vi "POST (File).vi"(6 "timeout":i32=10000, 7 "output file":path, 8 "error in":errorcluster, 9 "file":path, 10 "url":string, 11 "http-method in":refnum<class "REST Client.lvclass">) -> (0 "error out":errorcluster, 2 "response":refnum<class "response.lvclass">, 3 "http-method out":refnum<class "REST Client.lvclass">)   [LabVIEW 2020, in "REST Client.lvlib" / "REST Client.lvclass"]
uses:
  REST Client.lvclass
  response/response.lvclass
  http-client/http-client.lvclass
  REST Client.lvclass/REST Client.ctl
  http.lvlib
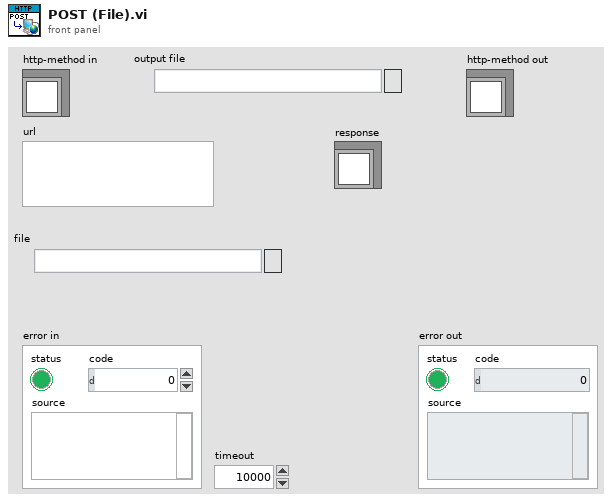
[diagram p1: front panel]
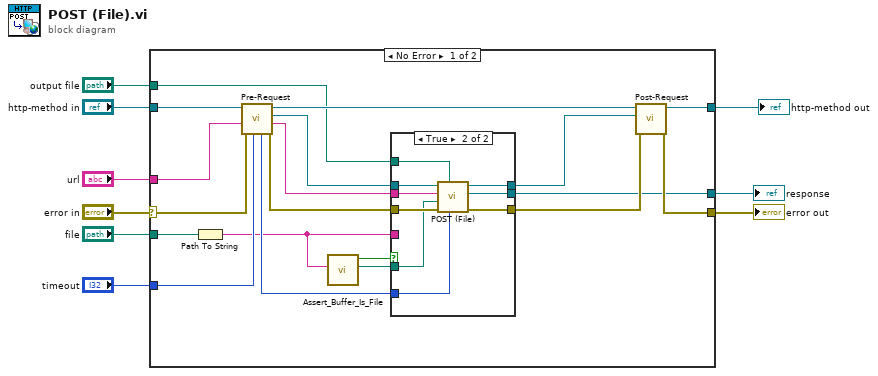
[diagram p0: block diagram]
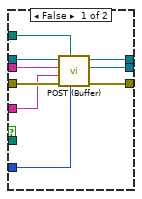
[diagram p2: hidden frame]
diagram:
  n1 = case shown="No Error" "error in" {
    selector: "error in" -> [w27 w48]
    tunnel: [w24 w48] -> w7
    tunnel: [w25 w47] -> w8
    tunnel: "http-method in" -> [w26 w47]
    tunnel: "url" -> [w22 _]
    tunnel: "timeout" -> [w21 _]
    tunnel: "output file" -> [w18 _]
    tunnel: "file" -> [w23 _]
    tunnel: [w10 _] -> w1
    frame No Error {
      n2 = Path To String(path=w23) -> (string=w14:string)
      n3 = call "Pre-Request.vi"("timeout"=w21, "error in (no error)"=w27, "url"=w22, "REST Client in"=w26) -> ("error out"=w16:errorcluster, "Resolved URL"=w13:string, "http-client"=w17:refnum<class "http-client.lvclass">, "REST Client out"=w28:refnum<class "REST Client.lvclass">, "Timeout"=w15:i32)  [unwired: 3 in]
      n4 = call "Assert_Buffer_Is_File.vi"("body"=w14) -> ("File"=w19:path, "is File?"=w20:bool)  [unwired: 9 in]
      n5 = case shown="True" w20 {
        tunnel: w19 -> [_ w38]
        tunnel: w14 -> [w33 _]
        tunnel: w17 -> [w37 w46]
        tunnel: w18 -> [w36 w45]
        tunnel: [w31 w44] -> w12
        tunnel: [w30 w43] -> w10
        tunnel: w15 -> [w29 w42]
        tunnel: w13 -> [w34 w41]
        tunnel: [w32 w40] -> w11
        tunnel: w16 -> [w35 w39]
        frame False {
          n6 = call-dynamic "POST (Buffer).vi"("timeout"=w29, "output file"=w36, "error in"=w35, "buffer"=w33, "url"=w34, "http-method in"=w37) -> ("error out"=w32:errorcluster, "response"=w30:refnum<class "response.lvclass">, "http-method out"=w31:refnum<class "http-client.lvclass">)  [unwired: 3 in]
        }
        frame True {
          n7 = call-dynamic "POST (File).vi"("timeout"=w42, "output file"=w45, "error in"=w39, "file"=w38, "url"=w41, "http-method in"=w46) -> ("error out"=w40:errorcluster, "REST Client.lvlib:response.lvclass"=w43:refnum<class "response.lvclass">, "http-method out"=w44:refnum<class "http-client.lvclass">)  [unwired: 3 in]
        }
      }
      n8 = call "Post-Request.vi"("error in (no error)"=w11, "http-method in"=w12, "REST Client in"=w28) -> ("error out"=w24:errorcluster, "REST Client out"=w25:refnum<class "REST Client.lvclass">)  [unwired: 7 in]
    }
    frame Error {
    }
  }
  "error out" <- w7
  "http-method out" <- w8
  "response" <- w1
